vi "Calculate Hold-In Voltage Measurements.vi"(0 "Stage Voltage Section":dbl[](array[numeric])) -> (4 "Max Stage":dbl, 6 "Min Stage":dbl, 8 "Avg Stage":dbl, 10 "Avg Max Stage":dbl, 14 "# of Pulses":dbl, 15 "Avg Min Stage":dbl)   [LabVIEW 2015, in "Fuel Injection Addon Engine.lvlib"]
uses:
  Fuel Injection Addon Engine.lvlib
  <vilib>/Analysis/baseanly.llb/Mean (DBL).vi
  <vilib>/Analysis/NI_AALBase.lvlib
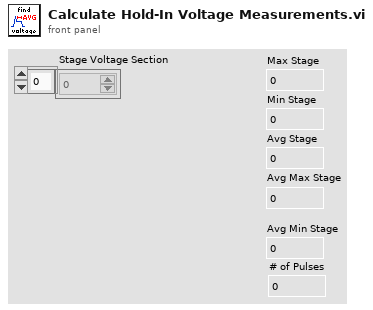
[diagram p1: front panel]
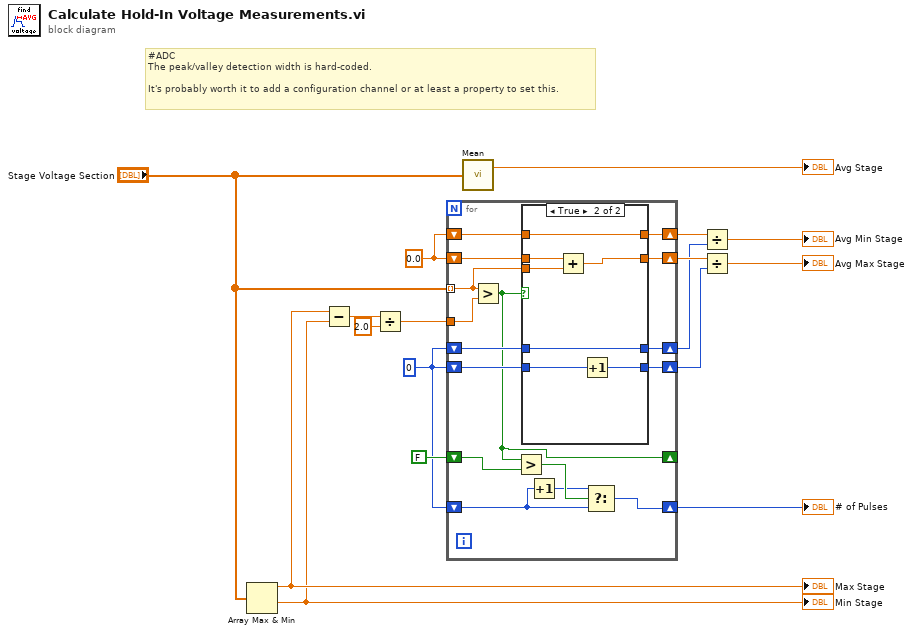
[diagram p0: block diagram]
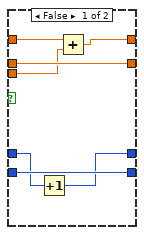
[diagram p2: hidden frame]
diagram:
  w2 = 0
  w7 = 0.0
  # "#ADC \nThe peak/valley detection width is hard-coded.\n\nIt's probably worth it to add a configuration channel or at least a property to set this."
  n1 = Array Max & Min(array="Stage Voltage Section") -> (max value=w16:dbl, min value=w15:dbl)  [unwired: 2 out]
  "Max Stage" <- w16
  "Min Stage" <- w15
  n2 = Subtract(x=w16, y=w15) -> (x-y=w14:dbl)
  n3 = Divide(x=w14, y=2.0) -> (x/y=w11:dbl)
  n4 = for {
    tunnel: "Stage Voltage Section" -> [w31] mode=indexing
    tunnel: w11 -> [w33]
    shift-right: [w30] -> w10
    shift-left: w7 -> [w32]
    shift-right: [w28] -> w9
    shift-left: w2 -> [w29]
    shift-right: [w26] -> w5
    shift-left: w2 -> [w27]
    shift-right: [w24] -> w6
    shift-left: w7 -> [w25]
    shift-right: [w18] -> _
    shift-left: FALSE -> [w23]
    shift-right: [w21] -> w1
    shift-left: w2 -> [w20]
    n5 = Greater?(x=w31, y=w33) -> (0:w18:bool)
    n6 = Greater?(x=w18, y=w23) -> (0:w22:bool)
    n7 = case shown="True" w18 {
      tunnel: w32 -> [w40 w47]
      tunnel: w31 -> [w35 w46]
      tunnel: [w40 w45] -> w30
      tunnel: w29 -> [w39 w44]
      tunnel: [w39 w43] -> w28
      tunnel: w27 -> [w38 w42]
      tunnel: [w37 w42] -> w26
      tunnel: w25 -> [w36 w41]
      tunnel: [w34 w41] -> w24
      frame False {
        n8 = Increment(x=w38) -> (x+1=w37:i32)
        n9 = Add(x=w36, y=w35) -> (x+y=w34:dbl)
      }
      frame True {
        n10 = Add(x=w47, y=w46) -> (x+y=w45:dbl)
        n11 = Increment(x=w44) -> (x+1=w43:i32)
      }
    }
    n12 = Increment(x=w20) -> (x+1=w19:i32)
    n13 = Select(t=w19, s=w22, f=w20) -> (s? t:f=w21:i32)
  }
  "# of Pulses" <- w1
  n14 = call-poly <vilib>:"Mean.vi"("X"="Stage Voltage Section") -> ("mean"=→"Avg Stage":dbl)  [unwired: 1 out]
  n15 = Divide(x=w6, y=w5) -> (x/y=→"Avg Min Stage":dbl)
  n16 = Divide(x=w10, y=w9) -> (x/y=→"Avg Max Stage":dbl)
